vi "MAIN.vi"() -> ()   [LabVIEW 2024]
uses:
  <vilib>/addons/database/Connection.llb/DB Tools Open Connec (Path).vi
  <vilib>/addons/database/_DB Variant To Data/Database Variant To Data.xnode
  <vilib>/addons/database/NI_Database_API.lvlib
panel:
  out "lowercase file extension":string
  out "indikator":T1
  in  "error in (no error) 4":errorcluster
  in  "error in (no error) 3":errorcluster
  in  "error in (no error) 2":errorcluster
  out "Array 4":string[](array[string])
  out "Array":string[](array[string])
  out "Array 3":i32[](array[numeric])
  out "Array 2":string[](array[string])
  out "x = y?":T1
  in  "error in (no error)":errorcluster
  out "error out":errorcluster
  in  "Tab Control":enum32{"Page 1", "Page 2", "Option"}(tab)
  in  "OK Button":bool
  in  "Next Button":bool
  in  "Foto":path
  in  "NIM":string
  in  "NAMA":string
  in  "Email":string
  in  "stop":bool
  out "new picture":picture
  in  "Ring":u16(ring) items=["PNG"=2, "JPEG"=1]
  in  "Previous Button":bool
  in  "Multicolumn Listbox":i32[](listbox)
  in  "Search":string
  in  "Search 2":bool
  in  "Email":string
  in  "Nama":string
  in  "NIM":string
  in  "Foto":path
  in  "update":bool
  in  "reset":bool
  in  "DELETE":bool
  out "new picture 2":picture
  in  "connection information":path
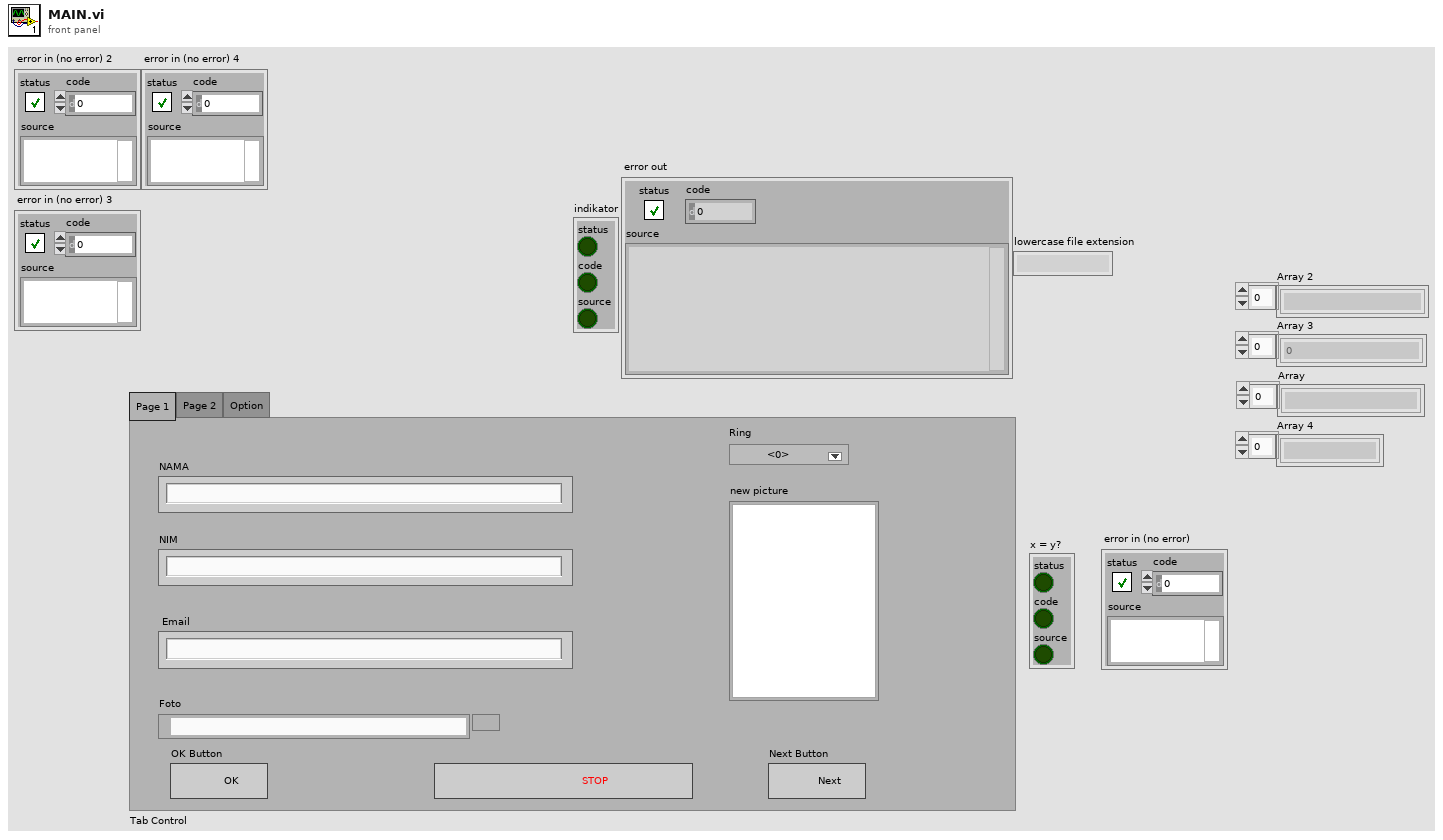
[diagram p1: front panel]
types:
  T1 = cluster{"status":bool, "code":bool, "source":bool}
  T2 = typedef "NI_Database_API.lvlib/Conn ObjectReference.ctl" = refnum<k1>
  T3 = typedef "imagedata.ctl" = cluster{"image type":i32, "image depth":i32, "image":u8[], "mask":u8[], "colors":u32[], "Rectangle":cluster{"left":i16, "top":i16, "right":i16, "bottom":i16}}
  T4 = typedef "LVBoundsTypeDef.ctl" = cluster{"Width":u32, "Height":u32}
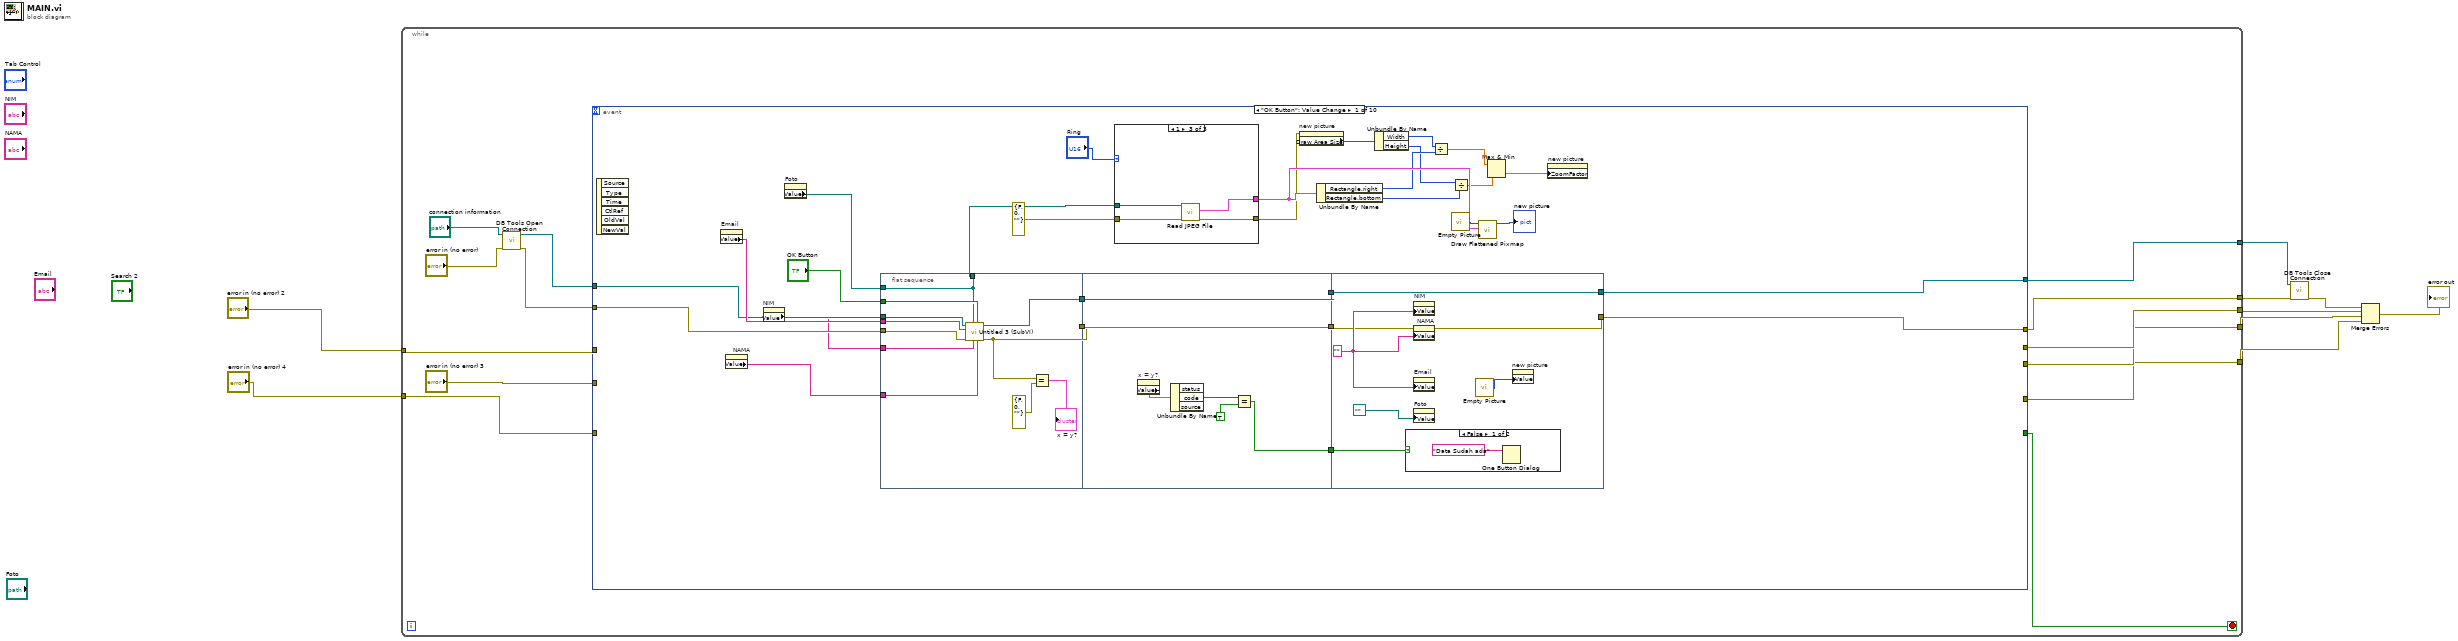
[diagram p0: block diagram]
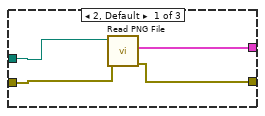
[diagram p2: hidden frame]
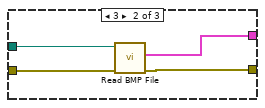
[diagram p3: hidden frame]
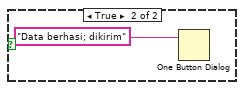
[diagram p4: hidden frame]
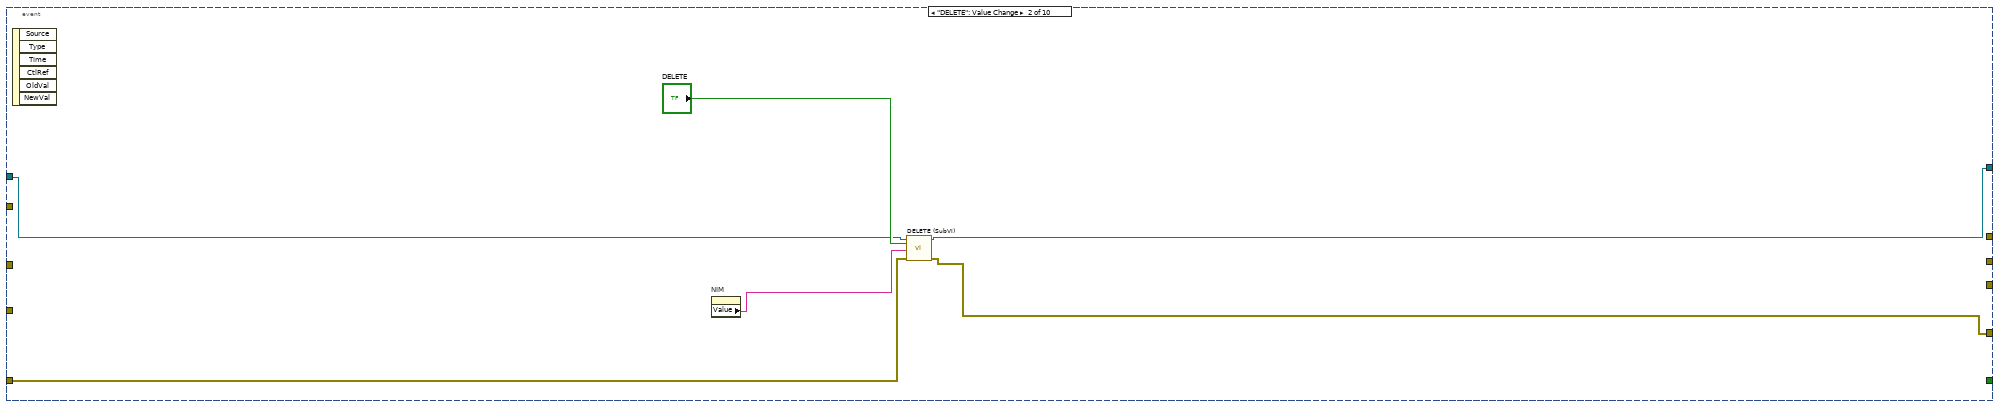
[diagram p5: hidden frame]
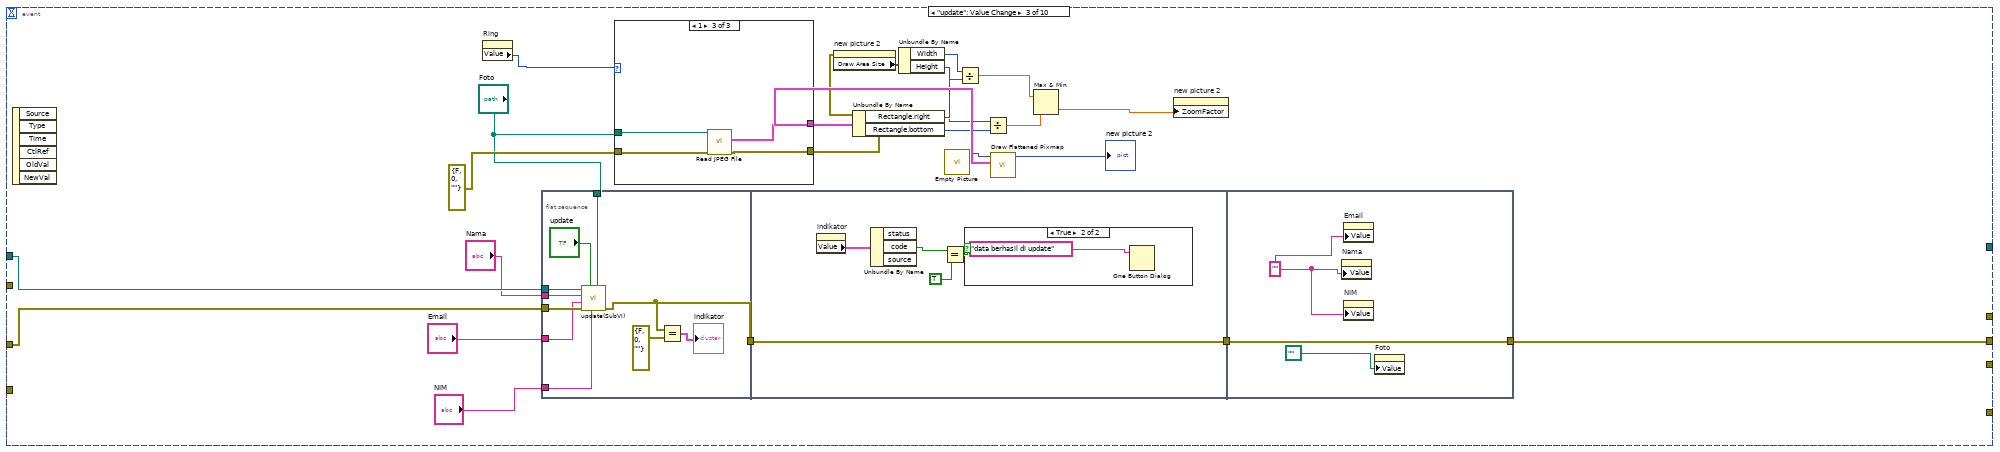
[diagram p6: hidden frame]
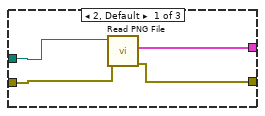
[diagram p7: hidden frame]
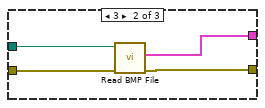
[diagram p8: hidden frame]
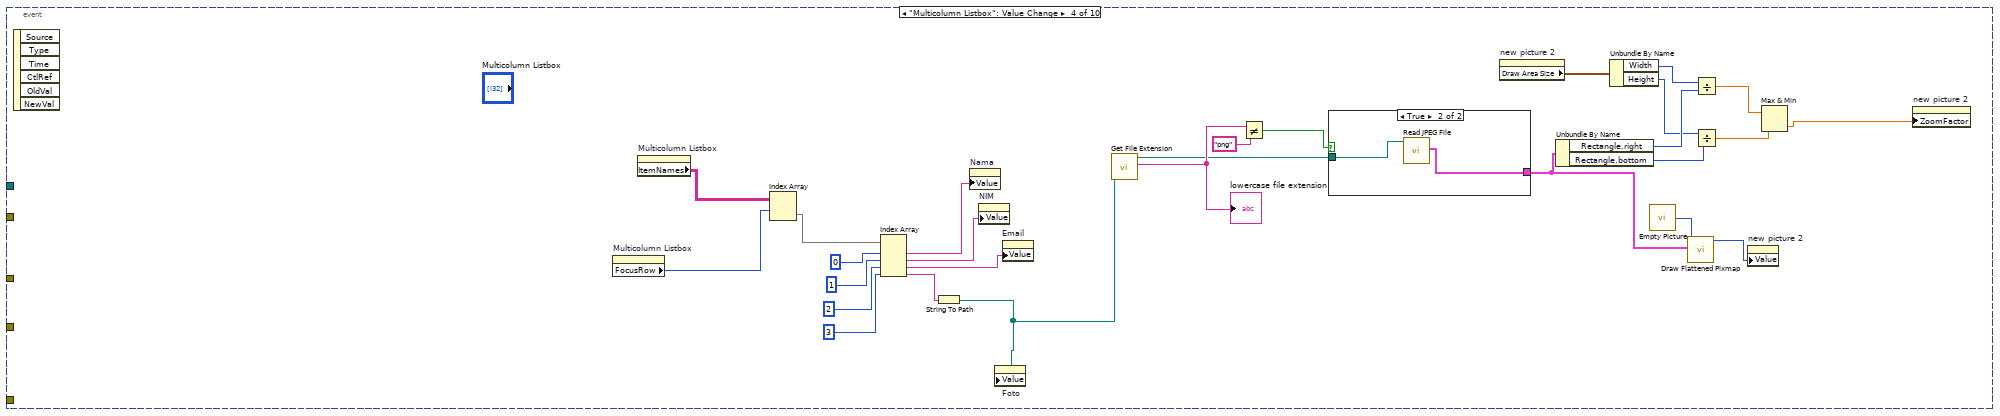
[diagram p10: hidden frame]
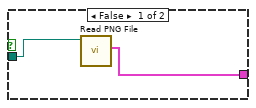
[diagram p11: hidden frame]
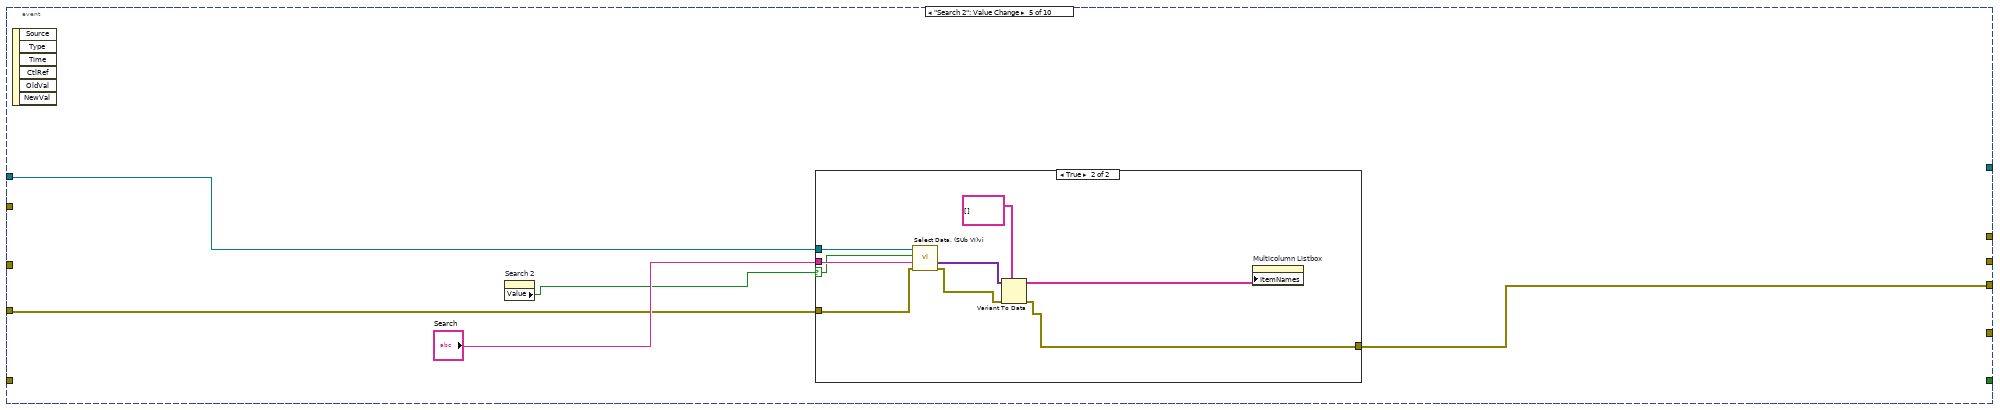
[diagram p12: hidden frame]
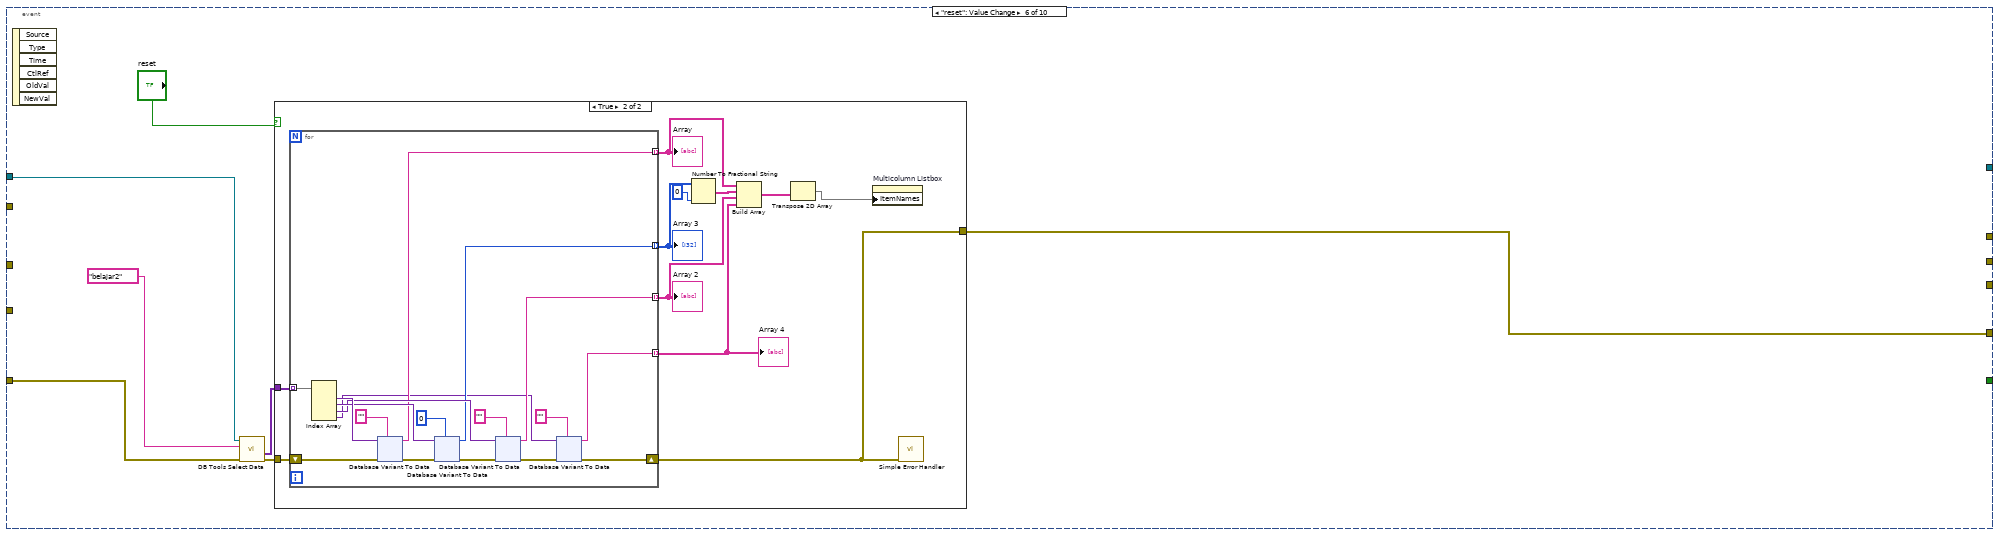
[diagram p14: hidden frame]
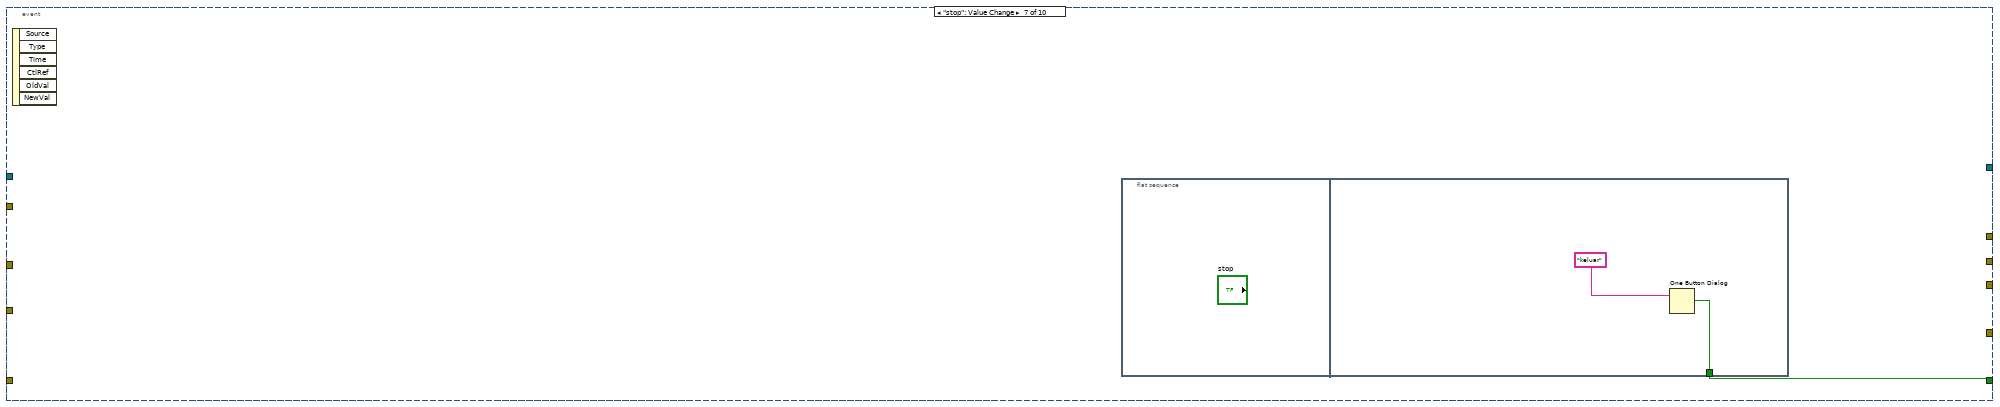
[diagram p16: hidden frame]
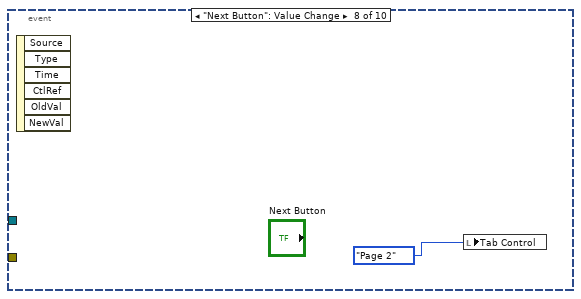
[diagram p17: hidden frame]
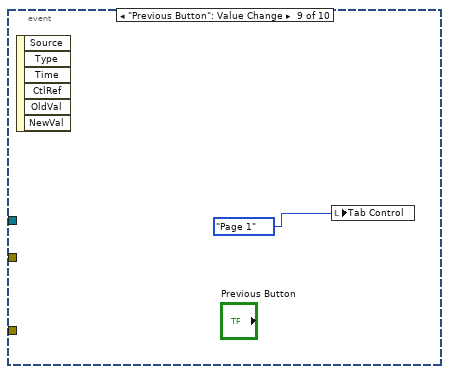
[diagram p18: hidden frame]
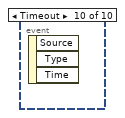
[diagram p19: hidden frame]
diagram:
  n1 = while {
    tunnel: [w21] -> w9
    tunnel: "error in (no error) 2" -> [w20]
    tunnel: [w19] -> w5
    tunnel: [w18] -> w4
    tunnel: [w17] -> w3
    tunnel: "error in (no error) 4" -> [w16]
    tunnel: [w14] -> w1
    stop <- w22 stop-if-true
    n2 = call-poly <vilib>:"DB Tools Open Connection.vi"("error in (no error)"="error in (no error)", "connection information"="connection information") -> ("error out"=w11:errorcluster, "connection reference"=w10:T2)  [unwired: 6 in]
    n3 = event shown="[0] \"OK Button\": Value Change" {
      selector: _ -> [_ _ _ _ _ _ _ _ _ _]
      dyn-events: _ -> [_ _ _ _ _ _ _ _ _ _]
      timeout: _ -> [_ _ _ _ _ _ _ _ _ _]
      tunnel: w10 -> [w49 w92 w117 _ w184 w198 _ _ _ _]
      tunnel: w20 -> [_ _ w116 _ _ _ _ _ _ _]
      tunnel: [_ _ _ _ _ _ w360 _ _ _] -> w22
      tunnel: [w48 _ _ _ _ _ _ _ _ _] -> w21
      tunnel: w11 -> [w47 _ _ _ _ _ _ _ _ _]
      tunnel: [_ _ w112 _ _ _ _ _ _ _] -> w19
      tunnel: "error in (no error) 3" -> [_ _ _ _ w182 _ _ _ _ _]
      tunnel: [_ _ _ _ w181 _ _ _ _ _] -> w18
      tunnel: [_ w90 _ _ _ w196 _ _ _ _] -> w17
      tunnel: w16 -> [_ w94 _ _ _ w195 _ _ _ _]
      tunnel: [w24 w91 _ _ _ _ _ _ _ _] -> w14
      event "OK Button": Value Change {
        n4 = event-data() -> ()  [unwired: 1 in, 6 out]
        n5 = property on="Email" class="Str"() -> ("Value"=w50:string)  [unwired: 2 in, 2 out]
        n6 = property on="NAMA" class="Str"() -> ("Value"=w51:string)  [unwired: 2 in, 2 out]
        n7 = property on="NIM" class="Str"() -> ("Value"=w46:string)  [unwired: 2 in, 2 out]
        n8 = property on="Foto" class="Path"() -> ("Value"=w25:path)  [unwired: 2 in, 2 out]
        n9 = flat-sequence {
          tunnel: w49 -> [w74]
          tunnel: w25 -> [w64]
          tunnel: w51 -> [w73]
          tunnel: w50 -> [w72]
          tunnel: w47 -> [w71]
          tunnel: w46 -> [w70]
          tunnel: [w68] -> w45
          tunnel: [w67] -> w43
          tunnel: "OK Button" -> [w65]
          tunnel: [w64] -> w23
          tunnel: w45 -> [w80]
          tunnel: [w80] -> w44
          tunnel: w43 -> [w79]
          tunnel: [w79] -> w42
          tunnel: [w75] -> w40
          tunnel: [w84] -> w48
          tunnel: w44 -> [w84]
          tunnel: w42 -> [w83]
          tunnel: [w83] -> w24
          tunnel: w40 -> [w82]
          frame #0 {
            n10 = call "Untitled 3 (SubVI).vi"("NIM"=w73, "Boolean"=w65, "Nama"=w70, "Foto"=w64, "error in (no error)"=w71, "Email"=w72, "Refnum in"=w74) -> ("error out"=w68:errorcluster, "Refnum out"=w67:T2)  [unwired: 2 in, 1 out]
            n11 = Equal?(x=w68, y=errorcluster {"status"=FALSE, "code"=0, "source"=""} ("error out")) -> (x = y?=→"x = y?":T1)
          }
          frame #1 {
            n12 = property on="x = y?" class="Clust (strict)"() -> ("Value"=w78:T1)  [unwired: 2 in, 2 out]
            n13 = Unbundle By Name(w78) -> ("code"=w77:bool)  [unwired: 2 out]
            n14 = Equal?(x=w77, y=TRUE) -> (x = y?=w75:bool)
          }
          frame #2 {
            w85 = ""
            n15 = case shown="False" w82 {
              frame False {
                n16 = One Button Dialog(message="Data Sudah ada") -> ()  [unwired: 1 in, 1 out]
              }
              frame True {
                n17 = One Button Dialog(message="Data berhasi; dikirim") -> ()  [unwired: 1 in, 1 out]
              }
            }
            n18 = property on="NIM" class="Str"("Value"=w85) -> ()  [unwired: 2 in, 2 out]
            n19 = property on="NAMA" class="Str"("Value"=w85) -> ()  [unwired: 2 in, 2 out]
            n20 = property on="Email" class="Str"("Value"=w85) -> ()  [unwired: 2 in, 2 out]
            n21 = property on="Foto" class="Path"("Value"=path "" ("Foto")) -> ()  [unwired: 2 in, 2 out]
            n22 = call "Empty Picture"() -> ("empty picture"=w81:picture)
            n23 = property on="new picture" class="Pict"("Value"=w81) -> ()  [unwired: 2 in, 2 out]
          }
        }
        n24 = case shown="1" "Ring" {
          tunnel: errorcluster {"status"=FALSE, "code"=0, "source"=""} ("error constant") -> [w55 w59 w63]
          tunnel: [w54 w58 w62] -> w34
          tunnel: w23 -> [w53 w57 w61]
          tunnel: [w52 w56 w60] -> w35
          frame 2, Default {
            n25 = call <vilib>:"Read PNG File.vi"("error in (no error)"=w55, "path to PNG file"=w53) -> ("error out"=w54:errorcluster, "image data"=w52:T3)  [unwired: 7 in, 1 out]
          }
          frame 3 {
            n26 = call <vilib>:"Read BMP File.vi"("error in (no error)"=w59, "path to BMP file"=w57) -> ("error out"=w58:errorcluster, "image data"=w56:T3)  [unwired: 7 in, 1 out]
          }
          frame 1 {
            n27 = call <vilib>:"Read JPEG File.vi"("error in (no error)"=w63, "path to JPEG file"=w61) -> ("error out"=w62:errorcluster, "image data"=w60:T3)  [unwired: 7 in, 1 out]
          }
        }
        n28 = property on="new picture" class="Pict"(error in=w34) -> ("Draw Area Size"=w33:T4)  [unwired: 1 in, 2 out]
        n29 = Unbundle By Name(w35) -> ("Rectangle.right"=w31:i16, "Rectangle.bottom"=w29:i16)
        n30 = Unbundle By Name(w33) -> ("Width"=w32:u32, "Height"=w30:u32)
        n31 = Divide(x=w32, y=w31) -> (x/y=w28:dbl)
        n32 = call "Empty Picture"() -> ("empty picture"=w36:picture)
        n33 = Divide(x=w30, y=w29) -> (x/y=w27:dbl)
        n34 = call <vilib>:"Draw Flattened Pixmap.vi"("image data"=w35, "picture"=w36) -> ("new picture"=→"new picture":picture)  [unwired: 7 in]
        n35 = Max & Min(x=w28, y=w27) -> (min(x,y)=w26:dbl)  [unwired: 1 out]
        n36 = property on="new picture" class="Pict"("ZoomFactor"=w26) -> ()  [unwired: 2 in, 2 out]
      }
      event "DELETE": Value Change {
        n37 = event-data() -> ()  [unwired: 1 in, 6 out]
        n38 = property on="NIM" class="Str"() -> ("Value"=w89:string)  [unwired: 2 in, 2 out]
        n39 = call "DELETE (SubVI).vi"("error in (no error)"=w94, "input 1"=w89, "Boolean"="DELETE", "Refnum in"=w92) -> ("error out"=w90:errorcluster, "Refnum out"=w91:T2)  [unwired: 6 in]
      }
      event "update": Value Change {
        n40 = event-data() -> ()  [unwired: 1 in, 6 out]
        n41 = property on="Ring" class="Ring (strict)"() -> ("Value"=w97:u16)  [unwired: 2 in, 2 out]
        n42 = flat-sequence {
          tunnel: w117 -> [w139]
          tunnel: w116 -> [w138]
          tunnel: "NIM" -> [w137]
          tunnel: "Nama" -> [w136]
          tunnel: "Email" -> [w135]
          tunnel: "Foto" -> [w134]
          tunnel: [w132] -> w111
          tunnel: w111 -> [w144]
          tunnel: [w144] -> w110
          tunnel: [w148] -> w112
          tunnel: w110 -> [w148]
          frame #0 {
            n43 = call "update(SubVI).vi"("Path"=w134, "nim"=w137, "Boolean"="update", "error in (no error)"=w138, "email"=w135, "nama"=w136, "Refnum in"=w139) -> ("error out"=w132:errorcluster)  [unwired: 2 in, 2 out]
            n44 = Equal?(x=w132, y=errorcluster {"status"=FALSE, "code"=0, "source"=""}) -> (x = y?=→"indikator":T1)
          }
          frame #1 {
            n45 = property on="indikator" class="Clust (strict)"() -> ("Value"=w143:T1)  [unwired: 2 in, 2 out]
            n46 = Unbundle By Name(w143) -> ("code"=w142:bool)  [unwired: 2 out]
            n47 = Equal?(x=w142, y=TRUE) -> (x = y?=w140:bool)
            n48 = case shown="True" w140 {
              frame False {
              }
              frame True {
                n49 = One Button Dialog(message="data berhasil di update") -> ()  [unwired: 1 in, 1 out]
              }
            }
          }
          frame #2 {
            w147 = ""
            n50 = property on="Nama" class="Str"("Value"=w147) -> ()  [unwired: 2 in, 2 out]
            n51 = property on="Email" class="Str"("Value"=w147) -> ()  [unwired: 2 in, 2 out]
            n52 = property on="NIM" class="Str"("Value"=w147) -> ()  [unwired: 2 in, 2 out]
            n53 = property on="Foto" class="Path"("Value"=path "" ("Foto")) -> ()  [unwired: 2 in, 2 out]
          }
        }
        n54 = case shown="1" w97 {
          tunnel: errorcluster {"status"=FALSE, "code"=0, "source"=""} ("error constant") -> [w121 w125 w129]
          tunnel: [w120 w124 w128] -> w98
          tunnel: "Foto" -> [w119 w123 w127]
          tunnel: [w118 w122 w126] -> w108
          frame 2, Default {
            n55 = call <vilib>:"Read PNG File.vi"("error in (no error)"=w121, "path to PNG file"=w119) -> ("error out"=w120:errorcluster, "image data"=w118:T3)  [unwired: 7 in, 1 out]
          }
          frame 3 {
            n56 = call <vilib>:"Read BMP File.vi"("error in (no error)"=w125, "path to BMP file"=w123) -> ("error out"=w124:errorcluster, "image data"=w122:T3)  [unwired: 7 in, 1 out]
          }
          frame 1 {
            n57 = call <vilib>:"Read JPEG File.vi"("error in (no error)"=w129, "path to JPEG file"=w127) -> ("error out"=w128:errorcluster, "image data"=w126:T3)  [unwired: 7 in, 1 out]
          }
        }
        n58 = property on="new picture 2" class="Pict"(error in=w98) -> ("Draw Area Size"=w99:T4)  [unwired: 1 in, 2 out]
        n59 = Unbundle By Name(w108) -> ("Rectangle.right"=w106:i16, "Rectangle.bottom"=w104:i16)
        n60 = Unbundle By Name(w99) -> ("Width"=w107:u32, "Height"=w105:u32)
        n61 = call "Empty Picture"() -> ("empty picture"=w101:picture)
        n62 = Divide(x=w107, y=w106) -> (x/y=w103:dbl)
        n63 = Divide(x=w105, y=w104) -> (x/y=w102:dbl)
        n64 = call <vilib>:"Draw Flattened Pixmap.vi"("image data"=w108, "picture"=w101) -> ("new picture"=→"new picture 2":picture)  [unwired: 7 in]
        n65 = Max & Min(x=w103, y=w102) -> (min(x,y)=w100:dbl)  [unwired: 1 out]
        n66 = property on="new picture 2" class="Pict"("ZoomFactor"=w100) -> ()  [unwired: 2 in, 2 out]
      }
      event "Multicolumn Listbox": Value Change {
        n67 = event-data() -> ()  [unwired: 1 in, 6 out]
        n68 = property on="Multicolumn Listbox" class="MCListbox (strict)"() -> ("FocusRow"=w174:i32)  [unwired: 2 in, 2 out]
        n69 = property on="Multicolumn Listbox" class="MCListbox (strict)"() -> ("ItemNames"=w175:string[][])  [unwired: 2 in, 2 out]
        n70 = Index Array(array=w175, index (row)=w174) -> (element=w173:string[])  [unwired: 1 in]
        n71 = Index Array(array=w173, index #1=0 ("index"), index #2=1 ("index"), index #3=2 ("index"), index #4=3 ("index")) -> (element #1=w168:string, element #2=w167:string, element #3=w166:string, element #4=w165:string)
        n72 = String To Path(string=w165) -> (path=w158:path)
        n73 = property on="Nama" class="Str"("Value"=w168) -> ()  [unwired: 2 in, 2 out]
        n74 = property on="NIM" class="Str"("Value"=w167) -> ()  [unwired: 2 in, 2 out]
        n75 = property on="Foto" class="Path"("Value"=w158) -> ()  [unwired: 2 in, 2 out]
        n76 = property on="Email" class="Str"("Value"=w166) -> ()  [unwired: 2 in, 2 out]
        n77 = call <vilib>:"Get File Extension.vi"("file"=w158) -> ("lowercase file extension"=w163:string, "dup file"=w162:path)  [unwired: 6 in, 3 out]
        "lowercase file extension" <- w163
        n78 = Not Equal?(x=w163, y="png") -> (x != y?=w164:bool)
        n79 = case shown="True" w164 {
          tunnel: w162 -> [w177 w179]
          tunnel: [w176 w178] -> w152
          frame False {
            n80 = call <vilib>:"Read PNG File.vi"("path to PNG file"=w177) -> ("image data"=w176:T3)  [unwired: 8 in, 2 out]
          }
          frame True {
            n81 = call <vilib>:"Read JPEG File.vi"("path to JPEG file"=w179) -> ("image data"=w178:T3)  [unwired: 8 in, 2 out]
          }
        }
        n82 = property on="new picture 2" class="Pict"() -> ("Draw Area Size"=w150:T4)  [unwired: 2 in, 2 out]
        n83 = Unbundle By Name(w152) -> ("Rectangle.right"=w156:i16, "Rectangle.bottom"=w151:i16)
        n84 = Unbundle By Name(w150) -> ("Width"=w157:u32, "Height"=w155:u32)
        n85 = call "Empty Picture"() -> ("empty picture"=w160:picture)
        n86 = call <vilib>:"Draw Flattened Pixmap.vi"("image data"=w152, "picture"=w160) -> ("new picture"=w159:picture)  [unwired: 7 in]
        n87 = Divide(x=w157, y=w156) -> (x/y=w154:dbl)
        n88 = Divide(x=w155, y=w151) -> (x/y=w153:dbl)
        n89 = property on="new picture 2" class="Pict"("Value"=w159) -> ()  [unwired: 2 in, 2 out]
        n90 = Max & Min(x=w154, y=w153) -> (min(x,y)=w149:dbl)  [unwired: 1 out]
        n91 = property on="new picture 2" class="Pict"("ZoomFactor"=w149) -> ()  [unwired: 2 in, 2 out]
      }
      event "Search 2": Value Change {
        n92 = event-data() -> ()  [unwired: 1 in, 6 out]
        n93 = property on="Search 2" class="Bool (strict)"() -> ("Value"=w180:bool)  [unwired: 2 in, 2 out]
        n94 = case shown="True" w180 {
          selector: w180 -> [_ w186]
          tunnel: w184 -> [_ w194]
          tunnel: "Search" -> [_ w193]
          tunnel: w182 -> [w185 w192]
          tunnel: [w185 w190] -> w181
          frame False {
          }
          frame True {
            n95 = call "Select Data. (SUb VI)vi.vi"("error in (no error)"=w192, "input 1"=w193, "Boolean"=w186, "Refnum in"=w194) -> ("error out 2"=w191:errorcluster, "recordset data"=w188:variant[][])  [unwired: 3 in, 3 out]
            n96 = Variant To Data(error in=w191, type=string[][] [], Variant=w188) -> (data=w187:string[][], error out=w190:errorcluster)
            n97 = property on="Multicolumn Listbox" class="MCListbox (strict)"("ItemNames"=w187) -> ()  [unwired: 2 in, 2 out]
          }
        }
      }
      event "reset": Value Change {
        n98 = event-data() -> ()  [unwired: 1 in, 6 out]
        n99 = call <vilib>:"DB Tools Select Data.vi"("error in (no error)"=w195, "table"="belajar2", "connection reference"=w198) -> ("error out"=w197:errorcluster, "data"=w200:variant[][])  [unwired: 3 in, 1 out]
        n100 = case shown="True" "reset" {
          tunnel: w200 -> [_ w207]
          tunnel: w197 -> [w202 w206]
          tunnel: [w202 w203] -> w196
          frame False {
          }
          frame True {
            n101 = for {
              shift-right: [w214] -> w203
              shift-left: w206 -> [w226]
              tunnel: [w223] -> w211 mode=indexing
              tunnel: [w221] -> w213 mode=indexing
              tunnel: [w220] -> w208 mode=indexing
              tunnel: w207 -> [w219] mode=indexing
              tunnel: [w215] -> w205 mode=indexing
              n102 = Index Array(array=w219) -> (element #1=w231:variant, element #2=w230:variant, element #3=w229:variant, element #4=w217:variant)  [unwired: 4 in]
              n103 = xnode "Database Variant To Data"("database variant"=w231, "error in (no error)"=w226, "type"="") -> ("data"=w220:string, "error out"=w225:errorcluster)
              n104 = xnode "Database Variant To Data"("database variant"=w230, "error in (no error)"=w225, "type"=0) -> ("data"=w221:i32, "error out"=w224:errorcluster)
              n105 = xnode "Database Variant To Data"("database variant"=w229, "error in (no error)"=w224, "type"="") -> ("data"=w223:string, "error out"=w218:errorcluster)
              n106 = xnode "Database Variant To Data"("database variant"=w217, "error in (no error)"=w218, "type"="") -> ("data"=w215:string, "error out"=w214:errorcluster)
            }
            "Array 2" <- w211
            "Array 3" <- w213
            "Array" <- w208
            "Array 4" <- w205
            n107 = Number To Fractional String(number=w213, precision (6)=i16 0) -> (F-format string=w212:string[])  [unwired: 2 in]
            n108 = Build Array(w208, w212, w211, w205) -> (w210:string[][])
            n109 = Transpose 2D Array(2D array=w210) -> (transposed array=w204:string[][])
            n110 = property on="Multicolumn Listbox" class="MCListbox (strict)"("ItemNames"=w204) -> ()  [unwired: 2 in, 2 out]
            n111 = call <vilib>:"Simple Error Handler.vi"("error in (no error)"=w203) -> ()  [unwired: 4 in, 5 out]
          }
        }
      }
      event "stop": Value Change {
        n112 = event-data() -> ()  [unwired: 1 in, 6 out]
        n113 = flat-sequence {
          tunnel: [w361] -> w360
          frame #0 {
          }
          frame #1 {
            n114 = One Button Dialog(message="keluar") -> (true=w361:bool)  [unwired: 1 in]
          }
        }
      }
      event "Next Button": Value Change {
        n115 = event-data() -> ()  [unwired: 1 in, 6 out]
        n116 = local write "Tab Control"(enum32{"Page 1", "Page 2"}."Page 2" ("Tab Control")) -> ()
      }
      event "Previous Button": Value Change {
        n117 = event-data() -> ()  [unwired: 1 in, 6 out]
        n118 = local write "Tab Control"(enum32{"Page 1", "Page 2"}."Page 1" ("Tab Control")) -> ()
      }
      event Timeout {
        n119 = event-data() -> ()  [unwired: 1 in, 3 out]
      }
    }
  }
  n120 = call <vilib>:"DB Tools Close Connection.vi"("error in (no error)"=w9, "connection reference"=w1) -> ("error out"=w7:errorcluster)  [unwired: 5 in]
  n121 = Merge Errors "Merge Errors"(w7, w5, w4, w3) -> (→"error out":errorcluster)
